vi "LVOOP DVR Access Snippet.vi"   [LabVIEW 2019]
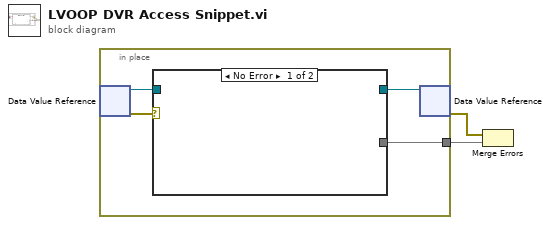
[diagram p0: block diagram]
diagram:
  n1 = in-place {
    in-place-border: [w4] -> w1
    n2 = in-place-dvr #1() -> (w5:refnum<class>, w6:errorcluster)  [unwired: 1 in]
    n3 = case shown="No Error" w6 {
      tunnel: w5 -> [_ w7]
      tunnel: [_ _] -> w4
      tunnel: [_ w7] -> w3
      frame No Error {
      }
      frame Error {
      }
    }
    n4 = in-place-dvr #1(w3) -> (w2:errorcluster)  [unwired: 1 out]
  }
  n5 = Merge Errors(w2, w1) -> ()  [unwired: 1 out]
